vi "TestLoadSingleimage.vi"() -> ()   [LabVIEW 2022 SP3]
uses:
  <userlib>/_OpenG.lib/file/file.llb/File Exists - Scalar__ogtk.vi
  <vilib>/vision/NI_Vision_Development_Module.lvlib
panel:
  out "error out 2":errorcluster
  out "File Type out":string
  out "error out":errorcluster
  in  "ImagePath":path
  out "ImageMain 3":T1(plugin-control)
  # "M:\\DigiLens-1276\\Printer Recipe Files\\Recipe_Patterns\\CalibrationPrints\\Strip Weights\\IP\\SW_IP1_0.bmp"
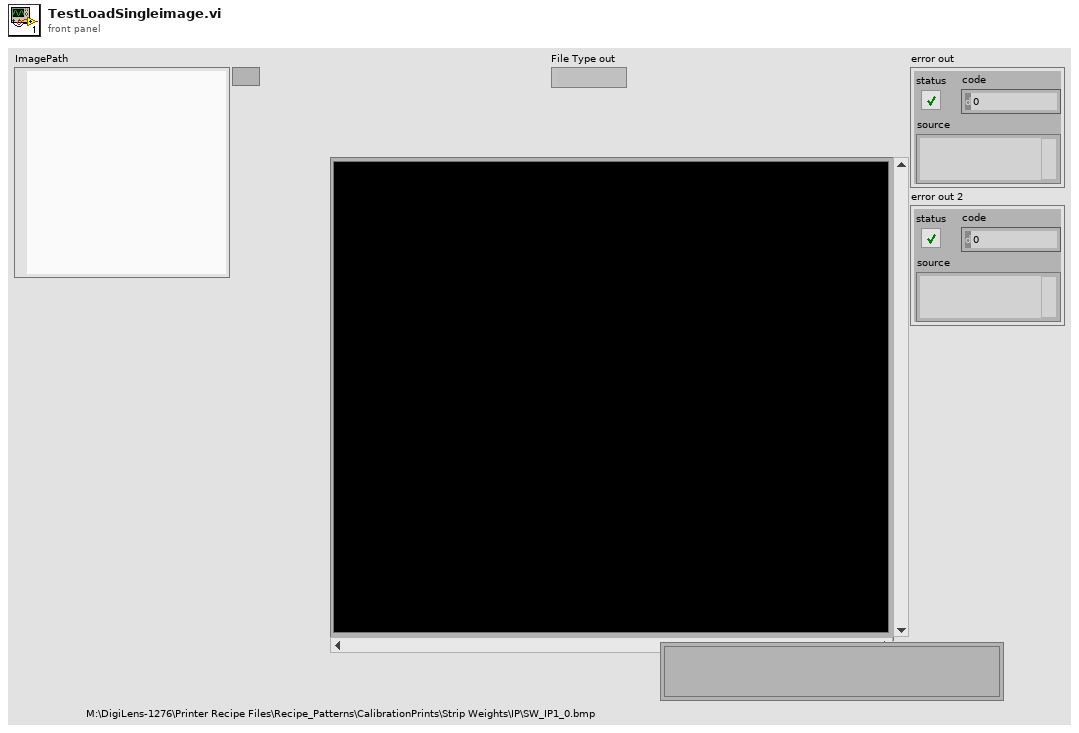
[diagram p1: front panel]
types:
  T1 = typedef "IMAQ Image.ctl" = refnum<image>
  T2 = typedef "Image Type" = u32
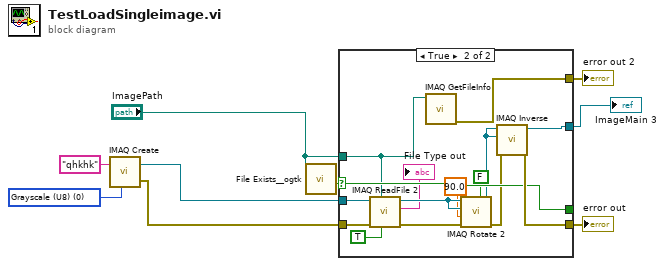
[diagram p0: block diagram]
diagram:
  w8 = T2 0 items=["Grayscale (U8)", "Grayscale (I16)", "Grayscale (SGL)", "Complex (CSG)", "RGB (U32)", "HSL (U32)", "RGB (U64)", "Grayscale (U16)"] ("Image Type")
  n1 = call "IMAQ Create"("Image Name"="qhkhk", "Image Type"=w8) -> ("New Image"=w7:T1, "error out"=w4:errorcluster)  [unwired: 3 in]
  n2 = call-poly <userlib>:"File Exists__ogtk.vi"("file path"="ImagePath") -> ("exists"=w6:bool)  [unwired: 6 in, 1 out]
  n3 = case shown="True" w6 {
    selector: w6 -> [w12 w23]
    tunnel: w7 -> [w11 w27]
    tunnel: [w10 w24] -> w3
    tunnel: [w11 w17] -> w2
    tunnel: "ImagePath" -> [_ w14]
    tunnel: [w12 w23] -> _
    tunnel: w4 -> [w10 w18]
    tunnel: [_ w13] -> w1
    frame False {
    }
    frame True {
      n4 = call "IMAQ ReadFile 2"("Use File Path Image Type"=TRUE, "File Path"=w14, "error in (no error)"=w18, "Image"=w27) -> ("error out"=w25:errorcluster, "File Type out"=→"File Type out":string, "Image Out"=w26:T1)  [unwired: 3 in, 2 out]
      n5 = call "IMAQ GetFileInfo"("File Path"=w14) -> ("error out"=w13:errorcluster)  [unwired: 4 in, 6 out]
      n6 = call "IMAQ Rotate 2"("Maintain Size"=FALSE, "error in (no error)"=w25, "Angle (degrees)"=90.0, "Image Dst"=w26, "Image Src"=w26) -> ("error out"=w20:errorcluster, "Image Dst Out"=w19:T1)  [unwired: 5 in]
      n7 = call "IMAQ Inverse"("error in (no error)"=w20, "Image Mask"=w19, "Image Src"=w19) -> ("error out"=w24:errorcluster, "Image Dst Out"=w17:T1)  [unwired: 7 in]
    }
  }
  "error out" <- w3
  "ImageMain 3" <- w2
  "error out 2" <- w1
